vi "LevelSelector.vi"(1 "Buttons":bool[](array[boolean])) -> (0 "Level":i32)   [LabVIEW 2014]
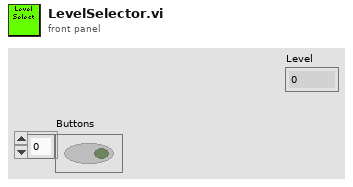
[diagram p1: front panel]
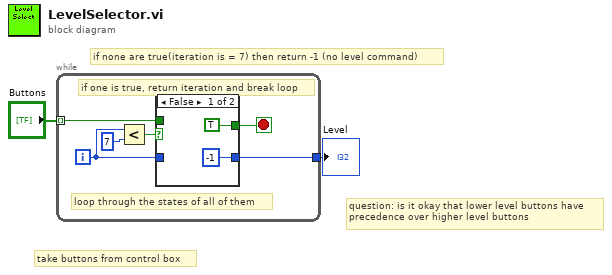
[diagram p0: block diagram]
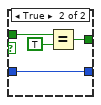
[diagram p2: hidden frame]
diagram:
  # "question: is it okay that lower level buttons have\nprecedence over higher level buttons"
  # "if none are true(iteration is = 7) then return -1 (no level command)"
  # "take buttons from control box"
  n1 = while {
    tunnel: "Buttons" -> [w8] mode=indexing
    tunnel: [w3] -> w1
    i -> [w4]
    stop <- w7 stop-if-true
    # "if one is true, return iteration and break loop"
    # "loop through the states of all of them"
    n2 = Less?(x=w4, y=7) -> (x < y?=w5:bool)
    n3 = case shown="False" w5 {
      tunnel: w8 -> [_ w14]
      tunnel: [TRUE w12] -> w7
      tunnel: w4 -> [_ w11]
      tunnel: [-1 w11] -> w3
      frame False {
      }
      frame True {
        n4 = Equal?(x=w14, y=TRUE) -> (x = y?=w12:bool)
      }
    }
  }
  "Level" <- w1
